vi "Draw.vi"(8 "error in (no error)":errorcluster, 11 "Selection in":refnum<class "Selection.lvclass">) -> (0 "error out":errorcluster, 2 "Picture":picture, 3 "Selection out":refnum<class "Selection.lvclass">)   [LabVIEW 2017, in "LV Image Editor Framework.lvlib" / "Selection.lvclass"]
uses:
  Selection.lvclass
  C:/Github/LIEF/Forms/Shape/Shape.lvclass
  Selection.lvclass/Selection.ctl
  Shape/Shape.lvclass
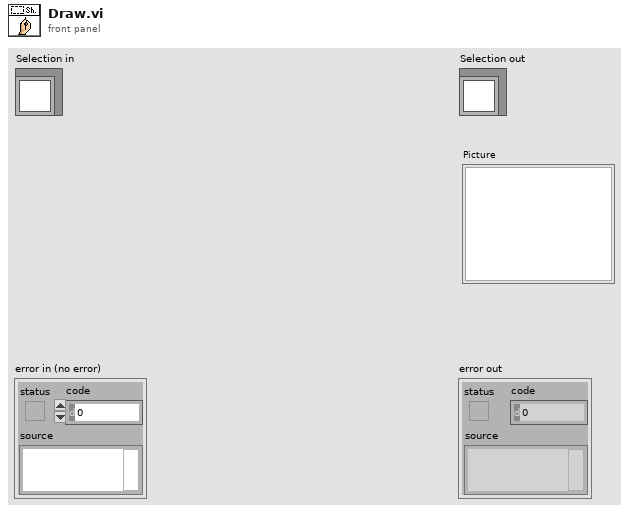
[diagram p1: front panel]
types:
  T1 = cluster{"Width":i16, "Style":enum32{"Solid", "Dash", "Dot", "DashDot", "DashDotDot"}}
  T2 = cluster{"Left":i32, "Top":i32, "Right":i32, "Bottom":i32}
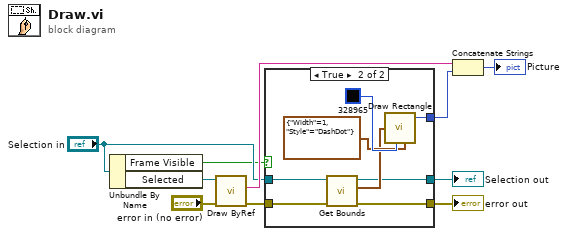
[diagram p0: block diagram]
diagram:
  n1 = Unbundle By Name("Selection in") -> ("Frame Visible"=w1:bool, "Selected"=w10:refnum<data-value>)
  n2 = call "Draw ByRef.vi"("error in (no error)"="error in (no error)", "ShapeRef"=w10) -> ("error out"=w6:errorcluster, "Raw Image"=w8:string)  [unwired: 7 in, 1 out]
  n3 = case shown="True" w1 {
    tunnel: [_ w17] -> w9
    tunnel: w6 -> [w11 w16]
    tunnel: "Selection in" -> [w12 w15]
    tunnel: [w11 w14] -> w3
    tunnel: [w12 w13] -> w2
    frame False {
    }
    frame True {
      n4 = call "Get Bounds.vi"("error in (no error)"=w16, "Shape in"=w15) -> ("error out"=w14:errorcluster, "Bounds"=w18:T2, "Shape out"=w13:refnum<class "Selection.lvclass">)  [unwired: 7 in]
      n5 = call <vilib>:"Draw Rectangle.vi"("rect"=w18, "color(black)"=u32 328965, "pen"=T1 {"Width"=1, "Style"=enum."DashDot"}) -> ("new picture"=w17:picture)  [unwired: 6 in]
    }
  }
  "error out" <- w3
  "Selection out" <- w2
  n6 = Concatenate Strings(w8, w9) -> (→"Picture":picture)
